vi "waveformChart.vi"() -> ()   [LabVIEW 2017]
panel:
  out "Waveform Chart":cluster{dbl, dbl}(graph)
  in  "stop":bool
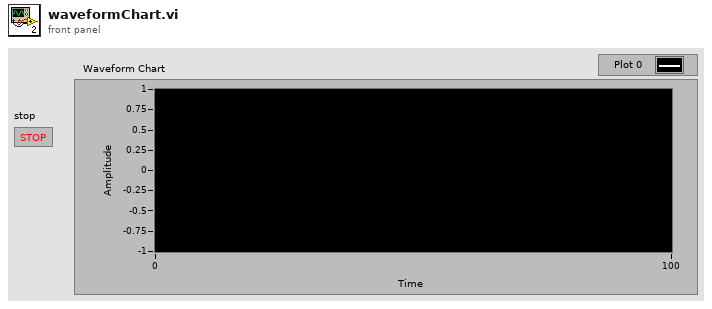
[diagram p1: front panel]
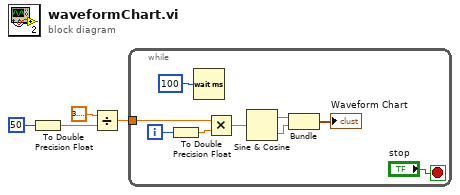
[diagram p0: block diagram]
diagram:
  n1 = To Double Precision Float(number=50) -> (double precision float=w1:dbl)
  n2 = Divide(x=3.141592653589793, y=w1) -> (x/y=w3:dbl)
  n3 = while {
    tunnel: w3 -> [w13]
    i -> [w10]
    stop <- "stop" stop-if-true
    n4 = To Double Precision Float(number=w10) -> (double precision float=w9:dbl)
    n5 = Wait (ms)(milliseconds to wait=100) -> ()  [unwired: 1 out]
    n6 = Multiply(x=w13, y=w9) -> (x*y=w8:dbl)
    n7 = Sine & Cosine(0:w8) -> (1:w7:dbl, 2:w6:dbl)
    n8 = Bundle(w7, w6) -> (→"Waveform Chart":cluster{dbl, dbl})  [unwired: 1 in]
  }
